vi "02 - Exemple - AsyncSum - DLL Call.vi"() -> ()   [LabVIEW 2016]
panel:
  in  "B":i32=2
  in  "A":i32=1
  out "Sum":i64
  # "+"
  # "="
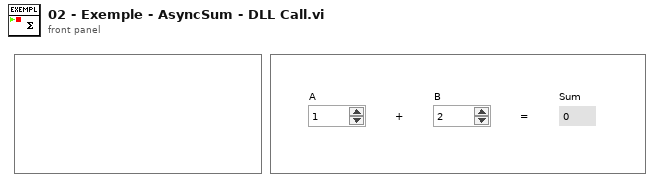
[diagram p1: front panel]
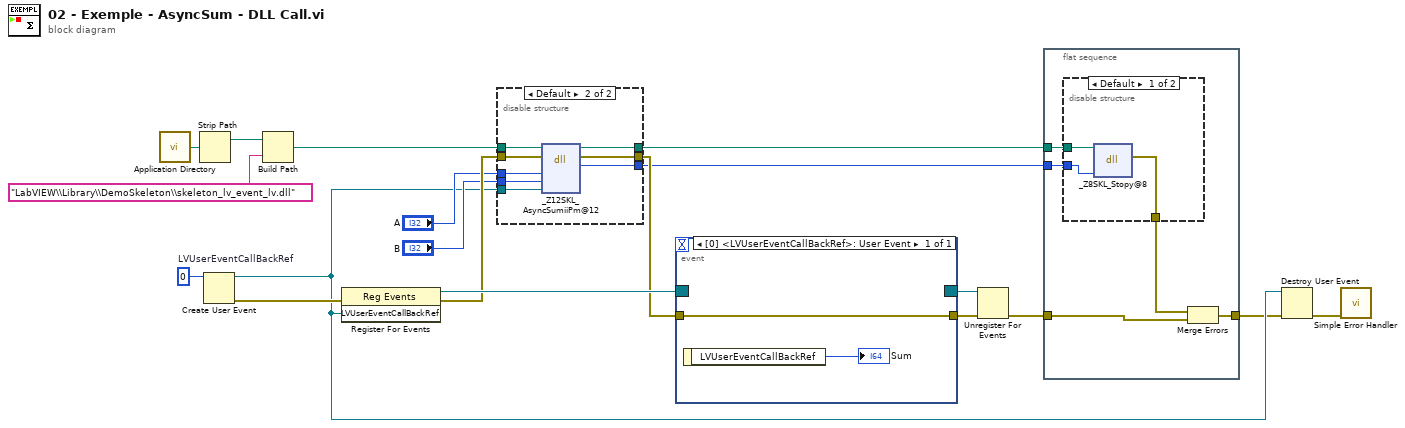
[diagram p0: block diagram]
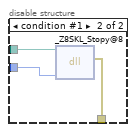
[diagram p2: hidden frame]
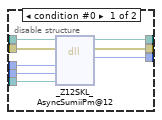
[diagram p3: hidden frame]
diagram:
  w14 = i64 0  # LVUserEventCallBackRef
  n1 = call <vilib>:"Application Directory.vi"() -> ("Application Directory"=w17:path)
  n2 = Strip Path(path=w17) -> (stripped path=w16:path)  [unwired: 1 out]
  n3 = Create User Event(user event datatype=w14) -> (user event=w6:refnum<user-event>, error out=w13:errorcluster)  [unwired: 1 in]
  n4 = Build Path(base path=w16, name or relative path="LabVIEW\\Library\\DemoSkeleton\\skeleton_lv_event_lv.dll") -> (appended path=w9:path)
  n5 = register-events(error in=w13, w6) -> (reference out=w12:refnum<event-registration>, error out=w11:errorcluster)  [unwired: 1 in]
  n6 = disable-structure shown="Default" {
    disable-tunnel: [w24 w33] -> w5
    disable-tunnel: w11 -> [w27 w35]
    disable-tunnel: [w25 w34] -> w10
    disable-tunnel: w6 -> [w26 w28]
    disable-tunnel: "A" -> [w23 w30]
    disable-tunnel: "B" -> [w22 w29]
    disable-tunnel: w9 -> [w21 w32]
    disable-tunnel: [w20 w31] -> w4
    frame condition #0 {
      n7 = dll-call lib="C:/Users/loic.wohleber/Desktop/PostLVUserEvent_Demo/Sources/LabVIEW/Library/DemoSkeleton/skeleton_lv_event_lvrt.dll" fn="_Z12SKL_AsyncSumiiPm@12" label="AsyncSum_RT"(path in=w21, error in=w27, "A"=w23, "B"=w22, "CallBackRefEvent"=w26) -> (path out=w20:path, error out=w25:errorcluster, "Handle"=w24:u64)  [unwired: 4 in]
    }
    frame condition #1 (active) {
      n8 = dll-call lib="C:/Users/loic.wohleber/Desktop/PostLVUserEvent_Demo/Sources/LabVIEW/Library/DemoSkeleton/skeleton_lv_event_lv.dll" fn="_Z12SKL_AsyncSumiiPm@12" label="AsyncSum"(path in=w32, error in=w35, "A"=w30, "B"=w29, "CallBackRefEvent"=w28) -> (path out=w31:path, error out=w34:errorcluster, "Handle"=w33:u64)  [unwired: 4 in]
    }
  }
  n9 = event shown="[0] <LVUserEventCallBackRef>: User Event" {
    selector: w12 -> [_]
    dyn-events: [_] -> w19
    timeout: _ -> [_]
    tunnel: w10 -> [w37]
    tunnel: [w37] -> w18
    event User Event {
      n10 = event-data() -> ("LVUserEventCallBackRef"=→"Sum":i64)  [unwired: 1 in]
    }
  }
  n11 = Unregister For Events(event registration refnum=w19, error in=w18) -> (error out=w3:errorcluster)
  n12 = flat-sequence {
    tunnel: w5 -> [w42]
    tunnel: w4 -> [w41]
    tunnel: w3 -> [w40]
    tunnel: [w38] -> w1
    frame #0 {
      n13 = disable-structure shown="Default" {
        disable-tunnel: [w45 w48] -> w39
        disable-tunnel: w42 -> [w43 w47]
        disable-tunnel: w41 -> [w44 w46]
        frame condition #0 (active) {
          n14 = dll-call lib="C:/Users/loic.wohleber/Desktop/PostLVUserEvent_Demo/Sources/LabVIEW/Library/DemoSkeleton/skeleton_lv_event_lv.dll" fn="_Z8SKL_Stopy@8" label="Stop"(path in=w44, "Handle"=w43) -> (error out=w45:errorcluster)  [unwired: 4 in, 1 out]
        }
        frame condition #1 {
          n15 = dll-call lib="C:/Users/loic.wohleber/Desktop/PostLVUserEvent_Demo/Sources/LabVIEW/Library/DemoSkeleton/skeleton_lv_event_lvrt.dll" fn="_Z8SKL_Stopy@8" label="StopRT"(path in=w46, "Handle"=w47) -> (error out=w48:errorcluster)  [unwired: 4 in, 1 out]
        }
      }
      n16 = Merge Errors(w39, w40) -> (w38:errorcluster)
    }
  }
  n17 = Destroy User Event(user event=w6, error in=w1) -> (error out=w2:errorcluster)
  n18 = call <vilib>:"Simple Error Handler.vi"("error in (no error)"=w2) -> ()  [unwired: 4 in, 5 out]
